vi "Write Trigger Core.vi"(8 "error in (no error)":errorcluster, 10 "PV":refnum<class "PV.lvclass">, 11 "DSConnection in":refnum<class "DSConnection.lvclass">) -> (0 "error out":errorcluster, 3 "DSConnection out":refnum<class "DSConnection.lvclass">)   [LabVIEW 2015, in "CS++ProcessVariables.lvlib" / "DSConnection.lvclass"]
doc: "Publish a process variable to trigger a paramater less message."
uses:
  DSConnection.lvclass
  ProcessVariable/PV.lvclass
  ProcessVariable/PV.lvclass/PV.ctl
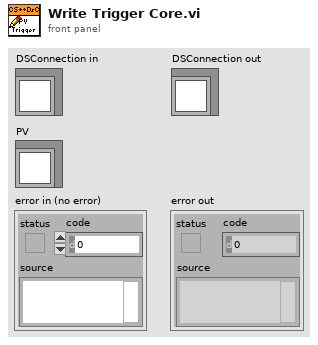
[diagram p1: front panel]
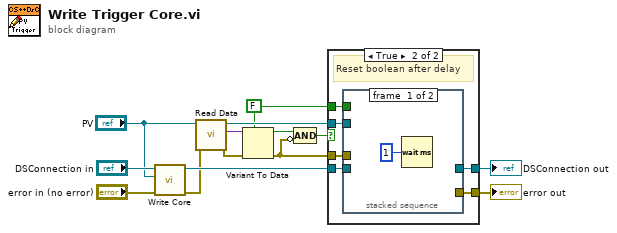
[diagram p0: block diagram]
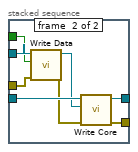
[diagram p3: hidden frame]
diagram:
  w7 = FALSE
  n1 = call-dynamic "Write Core.vi"("error in (no error)"="error in (no error)", "PV"="PV", "PVConnection in"="DSConnection in") -> ("error out"=w1:errorcluster, "PVConnection out"=w5:refnum<class "DSConnection.lvclass">)  [unwired: 7 in]
  n2 = call "Read Data.vi"("error in (no error)"=w1, "PV in"="PV") -> ("error out"=w11:errorcluster, "Data"=w10:variant, "PV out"=w8:refnum<class "PV.lvclass">)  [unwired: 7 in]
  n3 = Variant To Data(error in=w11, type=w7, Variant=w10) -> (data=w9:bool, error out=w6:errorcluster)
  n4 = Compound Arithmetic op=AND(w9, invert w6) -> (w2:bool)
  n5 = case shown="True" w2 {
    tunnel: w8 -> [_ w22]
    tunnel: w7 -> [_ w21]
    tunnel: w6 -> [w15 w20]
    tunnel: w5 -> [w16 w19]
    tunnel: [w16 w18] -> w4
    tunnel: [w15 w17] -> w3
    frame False {
    }
    frame True {
      # "Reset boolean after delay"
      n6 = stacked-sequence {
        tunnel: w22 -> [_ w31]
        tunnel: w21 -> [_ w30]
        tunnel: w20 -> [_ w29]
        tunnel: w19 -> [_ w28]
        tunnel: [_ w27] -> w18
        tunnel: [_ w24] -> w17
        frame #0 {
          n7 = Wait (ms)(milliseconds to wait=u32 1) -> ()  [unwired: 1 out]
        }
        frame #1 {
          n8 = call "Write Data.vi"("error in (no error)"=w29, "Data"=w30, "PV in"=w31) -> ("error out"=w26:errorcluster, "PV out"=w25:refnum<class "PV.lvclass">)  [unwired: 7 in]
          n9 = call-dynamic "Write Core.vi"("error in (no error)"=w26, "PV"=w25, "PVConnection in"=w28) -> ("error out"=w24:errorcluster, "PVConnection out"=w27:refnum<class "DSConnection.lvclass">)  [unwired: 7 in]
        }
      }
    }
  }
  "error out" <- w3
  "DSConnection out" <- w4
